vi "ChannelToneData_to_HDF5.vi"(0 "Timestamp":timestamp, 5 "ChannelToneData":T1={"Shift_"=0.0, "Peak_ToFPGA"=0.0, "MaxValue"=0.0, "MaxIndex"=0, "Tone"={"PkLocTrak"=0.0, "PkLocDisp"=0.0, "df_"=0.0, "ZoomPwr"=[], "Phase"=0.0, "PhaseOld"=0.0, "AboveThresh?"=FALSE, "MaxI"=0.0, "MaxQ"=0.0, "median"=0.0, "ISpect"=[], "QSpect"=[], "DeltaPhase"=0.0}, "TimeDomainI"=[], "TimeDomainQ"=[], "PwrSpectrum"=[], "RunningAvgFreq"=0.0, "ISpectPos"=[], "ISpectNeg"=[], "QSpectPos"=[], "QSpectNeg"=[], "10Hz_PwrSpectr"=[], "SNR"=0.0, "AliasWarn"=FALSE, "10Hz_Peak"=[], "ISpect+-"=[], "QSpect+-"=[], "TimeStamp"=timestamp(0 s since 1904-01-01), "I_Index"=array[12500 elements], "Q_Index"=array[12500 elements], "10MHz"=FALSE} {"Tone"."median" format="%0.2f"; "Tone"."MaxQ" format="%0.2f"}) -> (4 "Zoom":dbl[](array[numeric]), 6 "HDF5_ToneData":T3)   [LabVIEW 2018]
doc: "Convert Tone Data (either Beacon or Calibration) to clusters used for our HDF5 structure."
uses:
  HDF5_ToneInfoClust.ctl
  Controls/ToneInfoClust.ctl
  Controls/Clusts/ChannelToneData.ctl
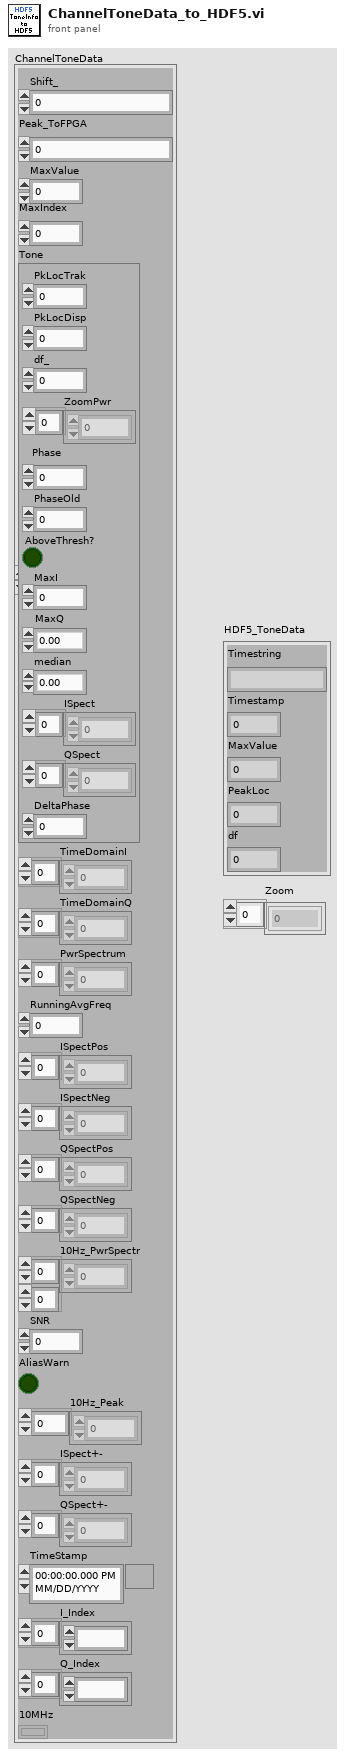
[diagram p1: front panel]
types:
  T1 = typedef "ChannelToneData.ctl" = cluster{"Shift_":dbl, "Peak_ToFPGA":dbl, "MaxValue":dbl, "MaxIndex":i32, "Tone":T2, "TimeDomainI":ext[], "TimeDomainQ":ext[], "PwrSpectrum":dbl[], "RunningAvgFreq":dbl, "ISpectPos":dbl[], "ISpectNeg":dbl[], "QSpectPos":dbl[], "QSpectNeg":dbl[], "10Hz_PwrSpectr":dbl[][], "SNR":dbl, "AliasWarn":bool, "10Hz_Peak":dbl[], "ISpect+-":dbl[], "QSpect+-":dbl[], "TimeStamp":timestamp, "I_Index":ext[], "Q_Index":ext[], "10MHz":bool}
  T2 = typedef "ToneInfoClust.ctl" = cluster{"PkLocTrak":dbl, "PkLocDisp":dbl, "df_":dbl, "ZoomPwr":dbl[], "Phase":dbl, "PhaseOld":dbl, "AboveThresh?":bool, "MaxI":dbl, "MaxQ":dbl, "median":dbl, "ISpect":dbl[], "QSpect":dbl[], "DeltaPhase":dbl}
  T3 = typedef "HDF5_ToneInfoClust.ctl" = cluster{"Timestring":string, "Timestamp":dbl, "MaxValue":dbl, "PeakLoc":dbl, "df":dbl}
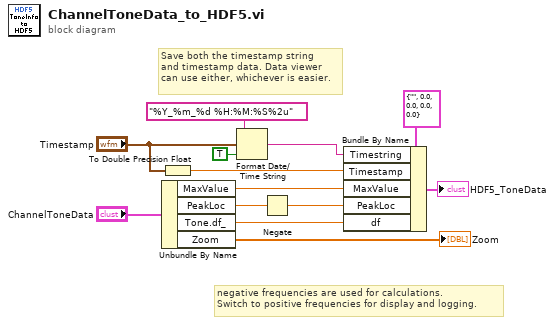
[diagram p0: block diagram]
diagram:
  # "negative frequencies are used for calculations.\nSwitch to positive frequencies for display and logging."
  # "Save both the timestamp string\nand timestamp data. Data viewer\ncan use either, whichever is easier."
  n1 = Unbundle By Name("ChannelToneData") -> ("MaxValue"=w7:dbl, "PeakLoc"=w8:dbl, "Tone.df_"=w9:dbl, "Zoom"=→"Zoom":dbl[])
  n2 = To Double Precision Float(number="Timestamp") -> (double precision float=w2:dbl)
  n3 = Format Date/Time String(time format string (%c)="%Y_%m_%d %H:%M:%S%2u", seconds (now)="Timestamp", UTC format=TRUE) -> (date/time string=w12:string)
  n4 = Negate(x=w8) -> (-x=w1:dbl)
  n5 = Bundle By Name(cluster=T3 {"Timestring"="", "Timestamp"=0.0, "MaxValue"=0.0, "PeakLoc"=0.0, "df"=0.0} ("HDF5_ToneInfo in"), "Timestring"=w12, "Timestamp"=w2, "MaxValue"=w7, "PeakLoc"=w1, "df"=w9) -> (→"HDF5_ToneData":T3)
